vi "Check Status (No Objects).vi"(8 "error in (no error)":errorcluster, 11 "Cluster In":T4={"Field"=0.0, "Rate"=0.0, "Status"={"Sweeping"=FALSE, "Clamped"=FALSE, "Hold"=FALSE, "At Rest"=FALSE, "Quench"=FALSE, "Persistent Mode"=FALSE, "Switch Heater"=FALSE}, "ILM Shut Down?"=FALSE, "IO Info"={"Address"={"Com Port"=1, "ISOBUS Address"=2, "GPIB Address"=24, "Communication"=enum."ISOBUS"}, "Version"=enum."IPS"}, "IO Info (Level Meter)"={"Address"={"Com Port"=1, "ISOBUS Address"=5, "GPIB Address"=24, "Communication"=enum."ISOBUS"}, "ILM Name"="", "Display Channel"=[]}, "Training?"=FALSE, "Training Field and Speed Cluster"={"Training Field"=[0.0, 4.108, 5.78, 8.001], "Training Speed"=[0.0057, 0.0022833333333333334, 0.0011333333333333334, 0.0011333333333333334]}}) -> (0 "error out":errorcluster, 1 "Status":string, 2 "Ready?":bool, 3 "Cluster Out":T4={"Field"=0.0, "Rate"=0.0, "Status"={"Sweeping"=FALSE, "Clamped"=FALSE, "Hold"=FALSE, "At Rest"=FALSE, "Quench"=FALSE, "Persistent Mode"=FALSE, "Switch Heater"=FALSE}, "ILM Shut Down?"=FALSE, "IO Info"={"Address"={"Com Port"=1, "ISOBUS Address"=2, "GPIB Address"=24, "Communication"=enum."ISOBUS"}, "Version"=enum."IPS"}, "IO Info (Level Meter)"={"Address"={"Com Port"=1, "ISOBUS Address"=5, "GPIB Address"=24, "Communication"=enum."ISOBUS"}, "ILM Name"="", "Display Channel"=[]}, "Training?"=FALSE, "Training Field and Speed Cluster"={"Training Field"=[0.0, 4.108, 5.78, 8.001], "Training Speed"=[0.0057, 0.0022833333333333334, 0.0011333333333333334, 0.0011333333333333334]}})   [LabVIEW 2017]
uses:
  Magnet status.ctl
  Oxford/PSSUBS.LLB/PSIO.ctl
  Oxford/BUSGEN.LLB/OxfordAddress.ctl
  Global/Relative Sound Files.vi
  Power Supply.lvclass
panel:
  out "approach0?":bool
  out "Field":dbl[unit]
  out "Field sweep rate":dbl[unit]
  out "switchheater":bool caption="Switch Heater"
  out "persis?":bool caption="Persistent Mode"
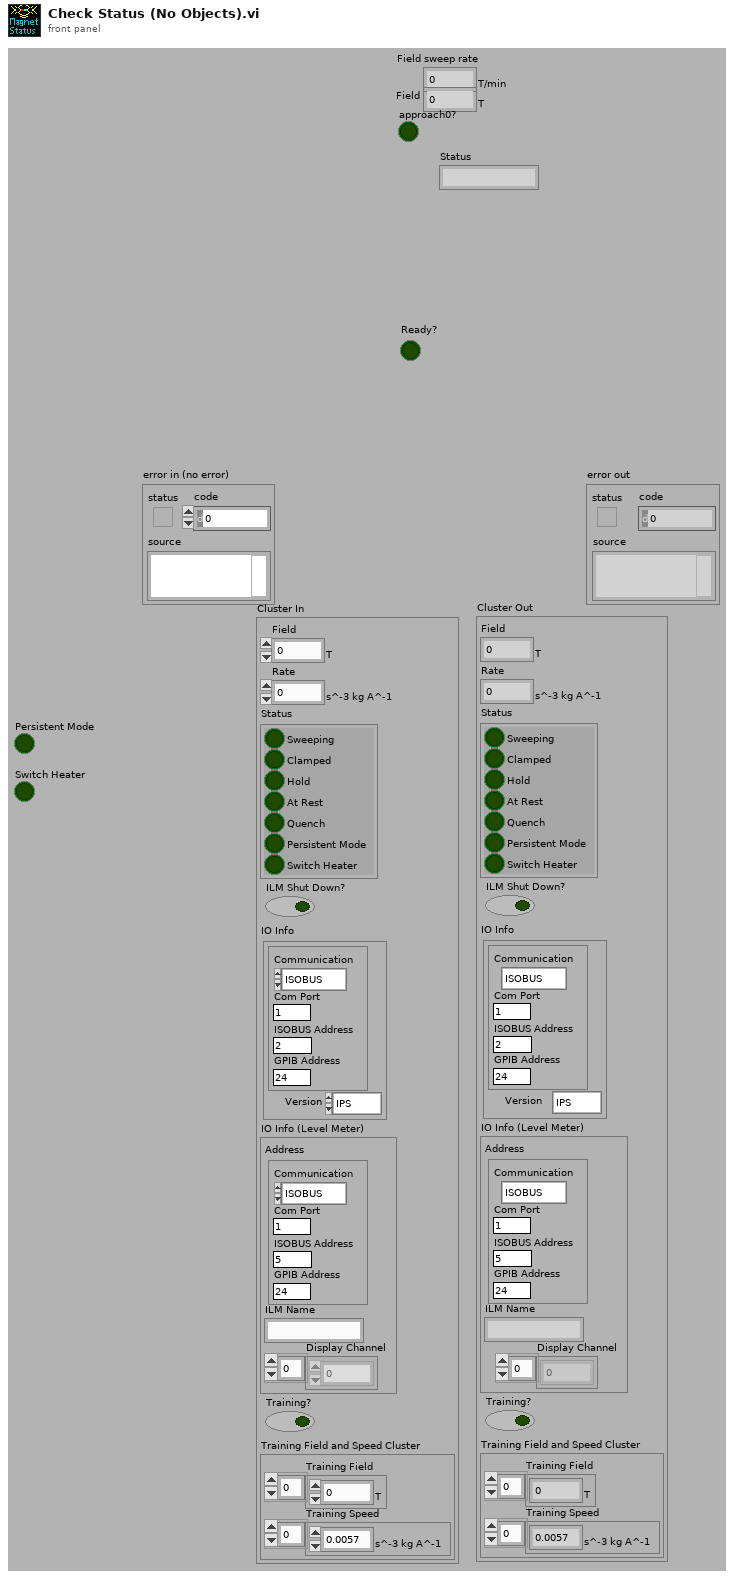
[diagram p1: front panel]
types:
  T1 = typedef "Power Supply.lvclass/Magnet status.ctl" = cluster{"Sweeping":bool, "Clamped":bool, "Hold":bool, "At Rest":bool, "Quench":bool, "Persistent Mode":bool, "Switch Heater":bool}
  T2 = typedef "PSIO.ctl" = cluster{"Address":T3, "Version":enum16{"PS", "IPS"}}
  T3 = typedef "OxfordAddress.ctl" = cluster{"Com Port":i32, "ISOBUS Address":i32, "GPIB Address":i16, "Communication":enum16{"RS232", "ISOBUS", "GPIB", "Gateway"}}
  T4 = cluster{"Field":dbl[unit], "Rate":dbl[unit], "Status":T1, "ILM Shut Down?":bool, "IO Info":T2, "IO Info (Level Meter)":cluster{"Address":T3, "ILM Name":string, "Display Channel":i32[]}, "Training?":bool, "Training Field and Speed Cluster":cluster{"Training Field":dbl[unit][], "Training Speed":dbl[unit][]}}
  T5 = typedef "ILMRelayStatus.ctl" = cluster{"Shut down":bool, "Alarm sound":bool, "Alarm state":bool, "Silence prohib":bool, "Relay1 active":bool, "Relay 2 active":bool, "Relay 3 active":bool, "Relay 4 active":bool}
  T6 = cluster{"Value":i16, "At rest":bool, "Sweeping":bool, "Rate limiting":bool}
  T7 = cluster{"Value":i16, "Hold":bool, "To set point":bool, "To zero":bool, "Clamped":bool}
  T8 = cluster{"Value":i16, "Off (at zero field)":bool, "On":bool, "Off (at field)":bool, "No switch fitted":bool, "Confirm":bool}
  T9 = cluster{"Value":i16, "Quenched":bool, "Over heated":bool, "Warming up":bool}
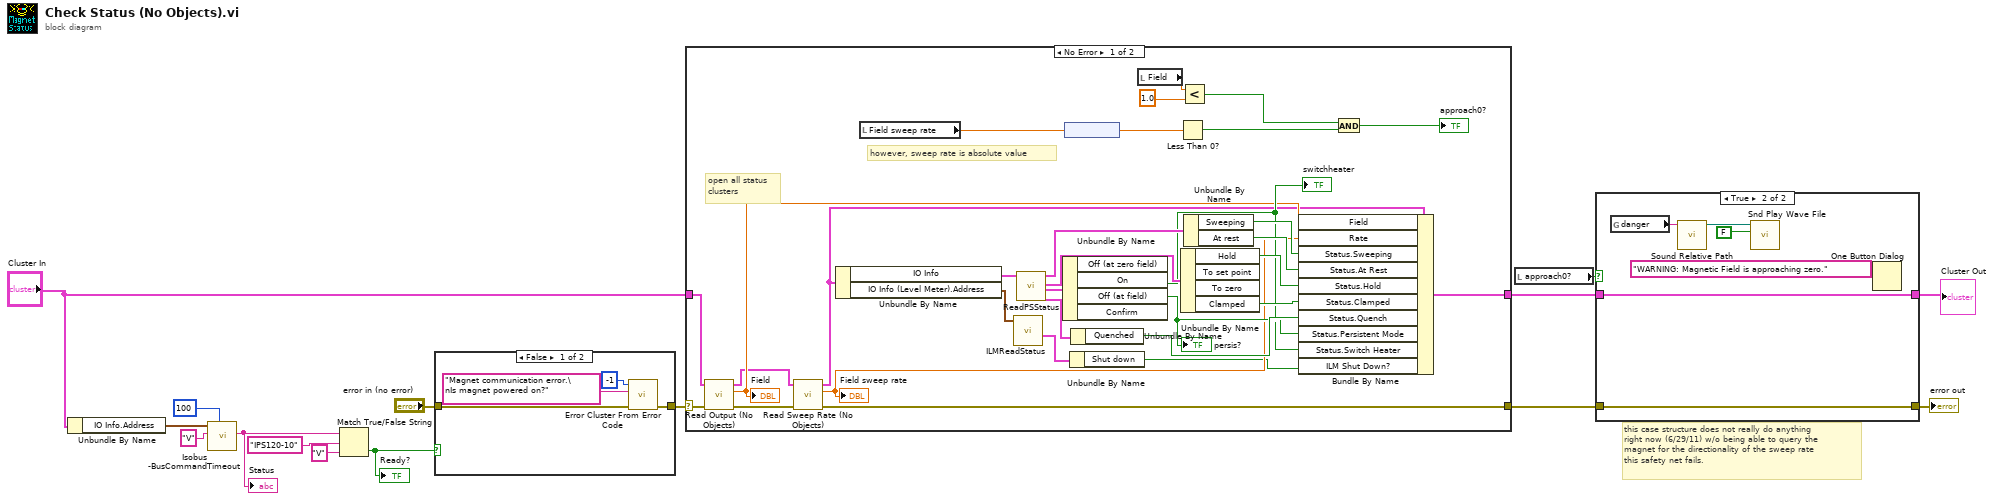
[diagram p0: block diagram]
diagram:
  # "this case structure does not really do anything\nright now (6/29/11) w/o being able to query the\nmagnet for the directionality of the sweep rate\nthis safety net fails."
  n1 = Unbundle By Name("Cluster In") -> ("IO Info.Address"=w11:T3)
  n2 = call "Isobus -BusCommandTimeout.vi"("Timeout (ms)"=100, "Command"="V", "Address"=w11) -> ("Reply"=w15:string)  [unwired: 5 out]
  "Status" <- w15
  n3 = Match True/False String(2:"V", 3:"IPS120-10", 4:w15) -> (0:w7:bool)  [unwired: 1 out]
  "Ready?" <- w7
  n4 = case shown="False" w7 {
    tunnel: "error in (no error)" -> [w17 w20]
    tunnel: [w16 w20] -> w8
    frame False {
      n5 = call <vilib>:"Error Cluster From Error Code.vi"("error in (no error)"=w17, "error message (\"\")"="Magnet communication error.\nIs magnet powered on?" ("error message (\"\")"), "error code (0)"=-1) -> ("error out"=w16:errorcluster)  [unwired: 6 in]
    }
    frame True {
    }
  }
  n6 = case shown="No Error" w8 {
    selector: w8 -> [w36 w52]
    tunnel: "Cluster In" -> [w22 w53]
    tunnel: [w38 w53] -> w6
    tunnel: [w35 w52] -> w5
    frame No Error {
      # "however, sweep rate is absolute value"
      # "open all status\nclusters"
      n7 = call "Read Output (No Objects).vi"("error in (no error)"=w36, "Cluster In"=w22) -> ("error out"=w37:errorcluster, "Field"=w40:dbl[unit], "Cluster Out"=w21:T4)  [unwired: 5 in, 2 out]
      "Field" <- w40
      n8 = call "Read Sweep Rate (No Objects).vi"("error in (no error)"=w37, "Cluster In"=w21) -> ("error out"=w35:errorcluster, "Field sweep rate"=w39:dbl[unit], "Cluster Out"=w34:T4)  [unwired: 7 in]
      "Field sweep rate" <- w39
      n9 = Unbundle By Name(w34) -> ("IO Info"=w33:T2, "IO Info (Level Meter).Address"=w25:T3)
      n10 = local read "Field sweep rate"() -> (w30:dbl[unit])
      n11 = call "ILMReadStatus.vi"("Instrument address"=w25) -> ("Relay"=w24:T5)  [unwired: 3 in, 3 out]
      n12 = call "ReadPSStatus.vi"("IO Info"=w33) -> ("Mode (n)"=w49:T6, "Activity"=w51:T7, "Switch Heater"=w50:T8, "System Status (m)"=w48:T9)  [unwired: 15 out]
      n13 = Unbundle By Name(w50) -> ("On"=w41:bool, "Off (at field)"=w42:bool)  [unwired: 2 out]
      "persis?" <- w42
      "switchheater" <- w41
      n14 = node(w30) -> (w29:dbl)
      n15 = Unbundle By Name(w24) -> ("Shut down"=w23:bool)
      n16 = Unbundle By Name(w48) -> ("Quenched"=w45:bool)
      n17 = local read "Field"() -> (w27:dbl[unit])
      n18 = Less Than 0?(x=w29) -> (x < 0?=w31:bool)
      n19 = Less?(x=w27, y=dbl[unit] 1.0) -> (x < y?=w32:bool)
      n20 = Unbundle By Name(w51) -> ("Hold"=w43:bool, "Clamped"=w46:bool)  [unwired: 2 out]
      n21 = Unbundle By Name(w49) -> ("Sweeping"=w47:bool, "At rest"=w44:bool)
      n22 = Bundle By Name(cluster=w34, "Field"=w40, "Rate"=w39, "Status.Sweeping"=w47, "Status.At Rest"=w44, "Status.Hold"=w43, "Status.Clamped"=w46, "Status.Quench"=w45, "Status.Persistent Mode"=w42, "Status.Switch Heater"=w41, "ILM Shut Down?"=w23) -> (w38:T4)
      n23 = And(x=w32, y=w31) -> (x .and. y?=→"approach0?":bool)
    }
    frame Error {
    }
  }
  n24 = local read "approach0?"() -> (w3:bool)
  n25 = case shown="True" w3 {
    tunnel: w6 -> [w55 w57]
    tunnel: w5 -> [w54 w58]
    tunnel: [w54 w58] -> w4
    tunnel: [w55 w57] -> w1
    frame False {
    }
    frame True {
      n26 = global read "Relative Sound Files.vi" "danger"() -> (w60:string)
      n27 = call "Sound Relative Path.vi"("Sound"=w60) -> ("Relative Path"=w59:path)  [unwired: 10 in]
      n28 = call <vilib>:"Snd Play Wave File.vi"("wait until finish (T)"=FALSE, "wave file path"=w59) -> ()  [unwired: 1 in, 9 out]
      n29 = One Button Dialog(message="WARNING: Magnetic Field is approaching zero.") -> ()  [unwired: 1 in, 1 out]
    }
  }
  "error out" <- w4
  "Cluster Out" <- w1
